vi "Get Steering Frame Bounds.vi"(8 "error in (no error)":errorcluster, 11 "steering frame in":refnum<class "NI_Robotics_Steering Frame.lvclass">) -> (0 "error out":errorcluster, 1 "length":dbl, 2 "width":dbl, 3 "steering frame out":refnum<class "NI_Robotics_Steering Frame.lvclass">, 4 "max dist from center":dbl, 6 "max wheel radius":dbl)   [LabVIEW 2017, in "NI_Robotics_Configure Steering Frame.lvlib"]
uses:
  <vilib>/robotics/Dialog/Configure Steering Frame/NI_Robotics_Configure Steering Frame.lvlib
  <vilib>/robotics/Steering/Steering Frame/NI_Robotics_Steering Frame.lvclass
  <vilib>/robotics/Steering/Steering Frame/NI_Robotics_Steering Frame.lvclass/NI_Robotics_Steering Frame.ctl
  <vilib>/robotics/Steering/Wheel/NI_Robotics_Wheel.lvclass/NI_Robotics_Wheel.ctl
  <vilib>/robotics/Steering/Steering Frame/Get Multiple Wheels in Steering Frame.vi
  <vilib>/robotics/Steering/Wheel/NI_Robotics_Wheel.lvclass
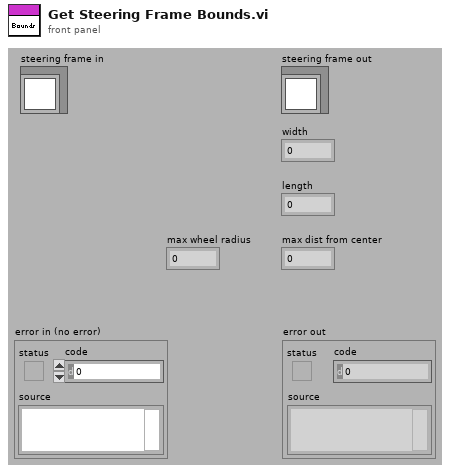
[diagram p1: front panel]
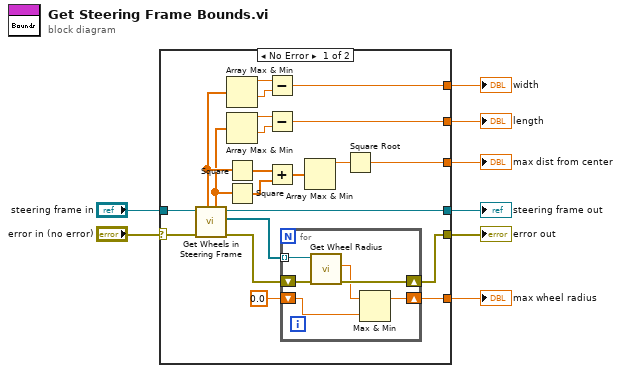
[diagram p0: block diagram]
diagram:
  n1 = case shown="No Error" "error in (no error)" {
    selector: "error in (no error)" -> [w28 w36]
    tunnel: "steering frame in" -> [w29 w37]
    tunnel: [w21 w37] -> w6
    tunnel: [w9 w36] -> w5
    tunnel: [w23 _] -> w4
    tunnel: [w22 _] -> w3
    tunnel: [w14 _] -> w2
    tunnel: [w11 _] -> w1
    frame No Error {
      n2 = call-poly <vilib>:"Get Wheels in Steering Frame.vi"("error in (no error)"=w28, "steering frame in"=w29) -> ("error out"=w10:errorcluster, "wheels"=w13:refnum<class "NI_Robotics_Wheel.lvclass">[], "steering frame out"=w21:refnum<class "NI_Robotics_Steering Frame.lvclass">, "y positions"=w19:dbl[], "x positions"=w20:dbl[])  [unwired: 3 in, 2 out]
      n3 = Array Max & Min(array=w20) -> (max value=w27:dbl, min value=w26:dbl)  [unwired: 2 out]
      n4 = Array Max & Min(array=w19) -> (max value=w25:dbl, min value=w24:dbl)  [unwired: 2 out]
      n5 = Square(x=w20) -> (x^2=w18:dbl[])
      n6 = Square(x=w19) -> (x^2=w17:dbl[])
      n7 = Subtract(x=w27, y=w26) -> (x-y=w23:dbl)
      n8 = Subtract(x=w25, y=w24) -> (x-y=w22:dbl)
      n9 = Add(x=w18, y=w17) -> (x+y=w16:dbl[])
      n10 = for {
        tunnel: w13 -> [w35] mode=indexing
        shift-right: [w33] -> w9
        shift-left: w10 -> [w34]
        shift-right: [w31] -> w11
        shift-left: 0.0 ("y") -> [w30]
        n11 = call <vilib>:"Get Wheel Radius.vi"("error in (no error)"=w34, "wheel in"=w35) -> ("error out"=w33:errorcluster, "wheel radius"=w32:dbl)  [unwired: 7 in, 1 out]
        n12 = Max & Min(x=w32, y=w30) -> (max(x,y)=w31:dbl)  [unwired: 1 out]
      }
      n13 = Array Max & Min(array=w16) -> (max value=w15:dbl)  [unwired: 3 out]
      n14 = Square Root(x=w15) -> (sqrt(x)=w14:dbl)
    }
    frame Error {
    }
  }
  "steering frame out" <- w6
  "error out" <- w5
  "width" <- w4
  "length" <- w3
  "max dist from center" <- w2
  "max wheel radius" <- w1
